vi "start_hil.vi"(4 "error in":errorcluster, 5 "Select a map":string(combo)="Almono", 6 "Scenario Configuration":path, 7 "Weather Profiles Ref":refnum<vi>) -> (0 "error out":errorcluster, 2 "Weather Profiles":T1(array[cluster]), 3 "Trajectory configuration":string)   [LabVIEW 2019]
doc: "Tool for initialization of a HIL mode program."
uses:
  controls/running_mode.ctl
  simx_common.vi
panel:
  in  "Simulator Configuration":string="{\n  \"id\": \"simulator\",\n  \"server_ip\": \"127.0.0.1\",\n  \"server_port\": 8999,\n  \"traffic_configuration\": {\n    \"max_vehicles\": 0,\n    \"min_desired_speed\": 0.0,\n    \"max_desired_speed\": 1.0,\n    \"spawn_leash_distance\": 15000,\n    \"min_spawn_range\": 2000,\n    \"swarm_traffic\": true,\n    \"vertical_offset\": 5,\n    \"overtake_slower_vehicles\" : false\n  },\n  \"phys_materials\": {\n    \"Aluminum\": {\n      \"specular_exponent\": 15.0,\n      \"specular_coefficient\": 0.95,\n      \"diffuse_coefficient\": 0.26,\n      \"dielectric_constant\": 10.0,\n      \"roughness\": 0.15\n    },\n    \"Asphalt\": {\n      \"specular_exponent\": 1.0,\n      \"specular_coefficient\": 0.03,\n      \"diffuse_coefficient\": 0.65,\n      \"dielectric_constant\": 7.0,\n      \"roughness\": 0.65\n    },\n    \"Road\": {\n      \"specular_exponent\": 1.0,\n      \"specular_coefficient\": 0.1,\n      \"diffuse_coefficient\": 0.65,\n      \"dielectric_constant\": 7.0,\n      \"roughness\": 0.65\n    },\n    \"Concrete\": {\n      \"specular_exponent\": 1.0,\n      \"specular_coefficient\": 0.0,\n      \"diffuse_coefficient\": 0.65,\n      \"dielectric_constant\": 7.0,\n      \"roughness\": 0.15\n    },\n    \"Glass\": {\n      \"specular_exponent\": 80.0,\n      \"specular_coefficient\": 0.80,\n      \"diffuse_coefficient\": 0.15,\n      \"dielectric_constant\": 4.0,\n      \"roughness\": 0.10\n    },\n    \"LandScape\": {\n      \"specular_exponent\": 10.0,\n      \"specular_coefficient\": 0.50,\n      \"diffuse_coefficient\": 0.50,\n      \"dielectric_constant\": 10.0,\n      \"roughness\": 0.60\n    },\n    \"Plastic\": {\n      \"specular_exponent\": 25.0,\n      \"specular_coefficient\": 0.40,\n      \"diffuse_coefficient\": 0.60,\n      \"dielectric_constant\": 2.8,\n      \"roughness\": 0.09\n    },\n    \"Steel\": {\n      \"specular_exponent\": 26.0,\n      \"specular_coefficient\": 1.0,\n      \"diffuse_coefficient\": 0.33,\n      \"dielectric_constant\": 0.0,\n      \"roughness\": 0.23\n    },\n    \"Tree\": {\n      \"specular_exponent\": 10.0,\n      \"specular_coefficient\": 0.05,\n      \"diffuse_coefficient\": 0.97,\n      \"dielectric_constant\": 10.0,\n      \"roughness\": 0.60\n    },\n    \"Wheel\": {\n      \"specular_exponent\": 92.0,\n      \"specular_coefficient\": 0.95,\n      \"diffuse_coefficient\": 0.06,\n      \"dielectric_constant\": 10.0,\n      \"roughness\": 0.15\n    },\n    \"Wood\": {\n      \"specular_exponent\": 10.0,\n      \"specular_coefficient\": 0.2,\n      \"diffuse_coefficient\": 0.7,\n      \"dielectric_constant\": 2.8,\n      \"roughness\": 0.80\n    },\n    \"Tire\": {\n      \"specular_exponent\": 25.0,\n      \"specular_coefficient\": 0.40,\n      \"diffuse_coefficient\": 0.60,\n      \"dielectric_constant\": 2.8,\n      \"roughness\": 0.15\n    }\n  },\n  \"simulation_mode\": 2,\n   \"map\": \"Almono\",\n  \"client_settings\": {\n    \"map\": {\n      \"gis_anchor\": { \"x\": 0, \"y\": 0, \"z\": 0},\n      \"point_delta\": 100.0\n    },\n    \"gui\":{\n      \"fps\": 1.0\n    },\n    \"logger\": {\n      \"sensor\": \"debug\",\n      \"network\": \"info\",\n      \"control\": \"info\",\n      \"scenario\": \"info\",\n      \"simulator\": \"info\",\n      \"vehicle\": \"info\"\n    }\n  }\n}"
  # "Change Setting for Simulator Configuration"
  # "DO NOT CHANGE"
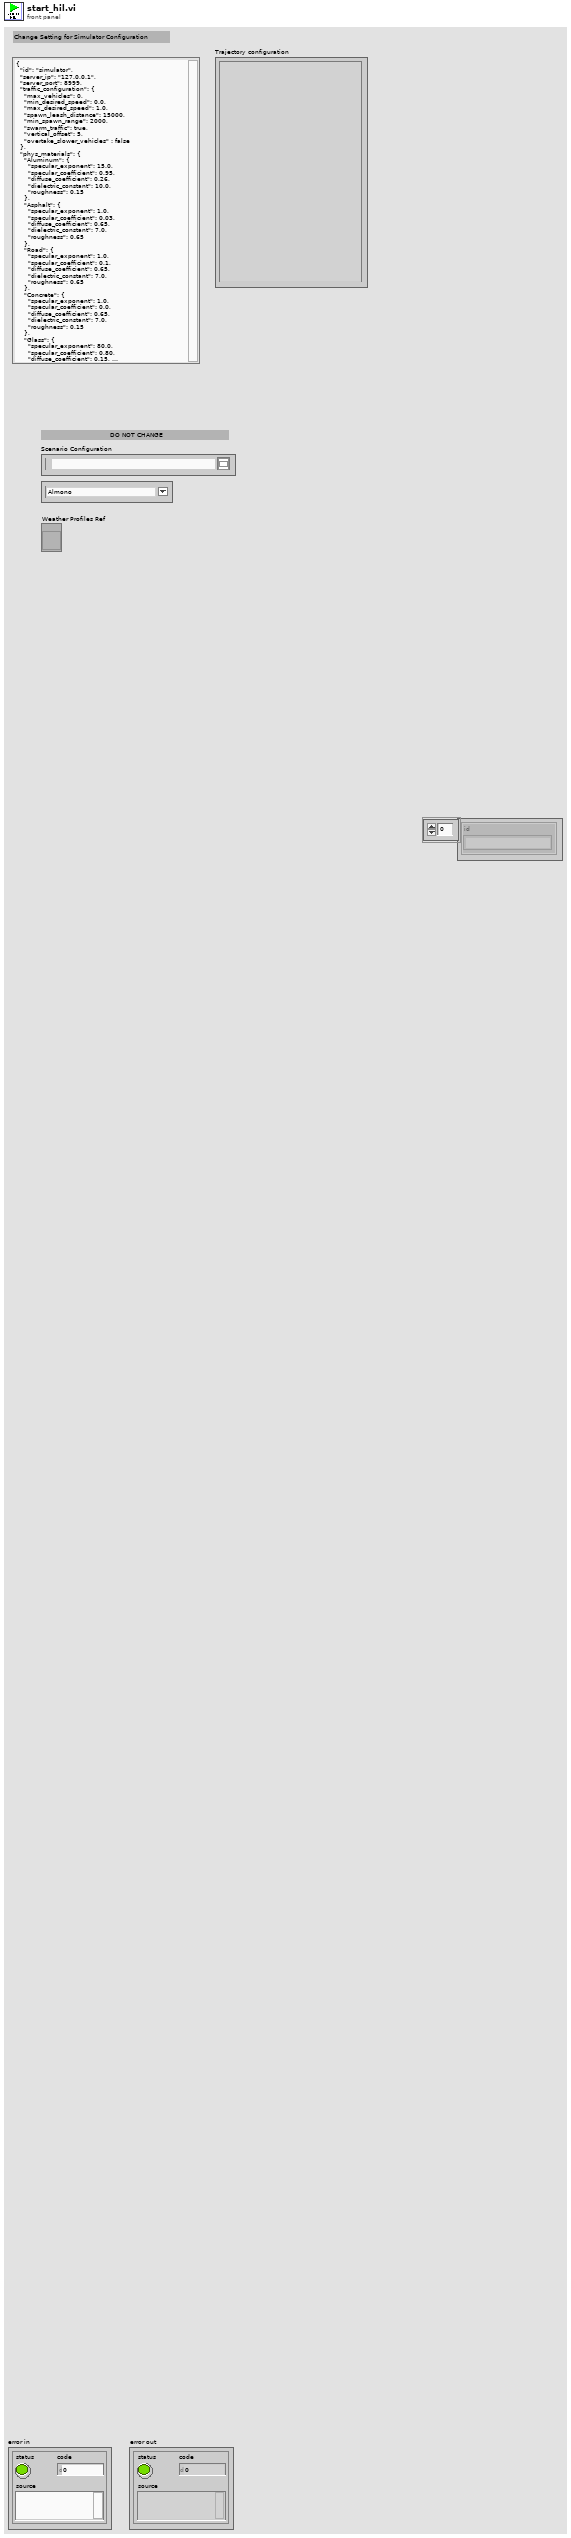
[diagram p1: front panel]
types:
  T1 = cluster{"id":string, "CloudColor":cluster{"A":sgl, "B":sgl, "G":sgl, "R":sgl}, "CloudOpacity":sgl, "Day":sgl, "FogCutoffDistance":sgl, "FogDensity":sgl, "FogHeightFalloff":sgl, "FogInscatteringColor":cluster{"A":sgl, "B":sgl, "G":sgl, "R":sgl}, "FogMaxOpacity":sgl, "FogStartDistance":sgl, "HorizonColor":cluster{"A":sgl, "B":sgl, "G":sgl, "R":sgl}, "HorizonFalloff":sgl, "Hours":sgl, "IsDaylightSavingTime":bool, "Latitude":sgl, "Longitude":sgl, "Minutes":sgl, "Month":sgl, "NorthOffset":sgl, "OverallSkyColor":cluster{"A":sgl, "B":sgl, "G":sgl, "R":sgl}, "OverideTimeBasedSunAngle":bool, "PrecipitationAccumulation":sgl, "PrecipitationAmount":sgl, "PrecipitationType":string, "SecondFogDensity":sgl, "SecondFogHeightFalloff":sgl, "SecondFogHeightOffset":sgl, "Seconds":sgl, "SkyLightColor":cluster{"A":sgl, "B":sgl, "G":sgl, "R":sgl}, "SkyLightIntensity":sgl, "StarBrightness":sgl, "SunAzimuthAngle":sgl, "SunBrightness":sgl, "SunDirectionalLightColor":cluster{"A":sgl, "B":sgl, "G":sgl, "R":sgl}, "SunDirectionalLightIntensity":sgl, "SunPolarAngle":sgl, "TimeZone":sgl, "WindAngle":sgl, "WindIntensity":sgl, "Year":sgl, "ZenithColor":cluster{"A":sgl, "B":sgl, "G":sgl, "R":sgl}, "bPrecipitation":bool, "bWind":bool}[]
  T2 = typedef "running_mode.ctl" = i32
  T3 = typedef "simx_connection.ctl" = cluster{"Config":T4, "Connections":T7, "Map":cluster{"lanes":cluster{"x":dbl[], "y":dbl[], "z":dbl[]}, "StartPosition":cluster{"start_points":T8, "StartRotation":dbl[], "StartLocation":dbl[]}, "Draw Map Size":T9, "DrawArea":cluster{"min_Y":dbl, "min_X":dbl, "Scale X":dbl, "Scale Y":dbl}, "Map":picture, "Map Geojson":string}}
  T4 = typedef "config.ctl" = cluster{"Trajectory":T5, "Weather":T6}
  T5 = typedef "trajectory.ctl" = cluster{"Number of frames":i32, "Frame number":i32, "Trajectory":string}
  T6 = typedef "weather.ctl" = cluster{"id":string}
  T7 = typedef "connections.ctl" = cluster{"Simulator Connection":refnum<k5>, "server_ip":string, "Port":i32, "Sensor connections":refnum<k5>[]}
  T8 = typedef "start_points.ctl" = cluster{"locations":dbl[][], "rotations":dbl[][], "type":string[]}
  T9 = typedef "LVBoundsTypeDef.ctl" = cluster{"Width":u32, "Height":u32}
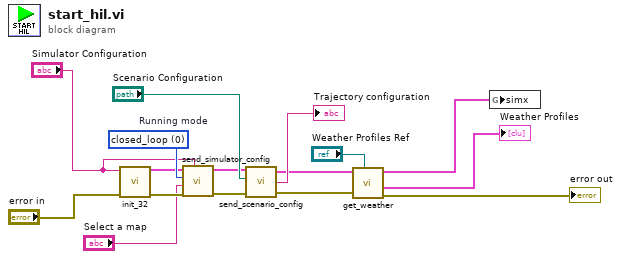
[diagram p0: block diagram]
diagram:
  w15 = T2 0 items=["closed_loop", "replay", "hil"]  # Running mode
  n1 = call "init_32.vi"("error in"="error in", "Simulator Configuration"="Simulator Configuration") -> ("error out"=w7:errorcluster, "simx out"=w6:T3)  [unwired: 4 in]
  n2 = call "send_simulator_config.vi"("Simulator Configuration"="Simulator Configuration", "error in"=w7, "Select a map"="Select a map", "Running mode"=w15, "simx in"=w6) -> ("error out"=w5:errorcluster, "monoDrive out"=w4:T3)  [unwired: 2 in]
  n3 = call "send_scenario_config.vi"("simx in"=w4, "Scenario Configuration"="Scenario Configuration", "error in"=w5) -> ("simx out"=w9:T3, "Scenario configuration"=→"Trajectory configuration":string, "error out"=w8:errorcluster)  [unwired: 3 in]
  n4 = call "get_weather.vi"("Weather Profiles"="Weather Profiles Ref", "error in"=w8, "simx in"=w9) -> ("error out"=→"error out":errorcluster, "Weather Profiles"=→"Weather Profiles":T1, "simx out"=w3:T3)  [unwired: 3 in, 1 out]
  n5 = global write "simx_common.vi" "simx"(w3) -> ()
